vi "Motors Sub 05.vi"(7 "Cluster":T1, 8 "error in":errorcluster, 11 "VISA in":refnum<visa-resource-name>) -> (0 "error out":errorcluster, 3 "VISA out":refnum<visa-resource-name>)   [LabVIEW 2010]
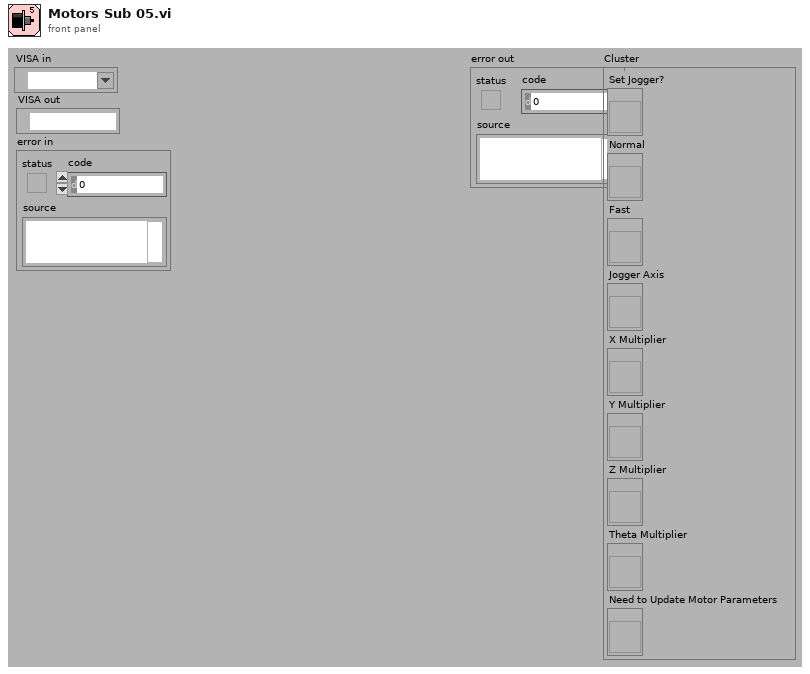
[diagram p1: front panel]
types:
  T1 = cluster{"Set Jogger?":refnum<vi>, "Normal":refnum<vi>, "Fast":refnum<vi>, "Jogger Axis":refnum<vi>, "X Multiplier":refnum<vi>, "Y Multiplier":refnum<vi>, "Z Multiplier":refnum<vi>, "Theta Multiplier":refnum<vi>, "Need to Update Motor Parameters":refnum<vi>}
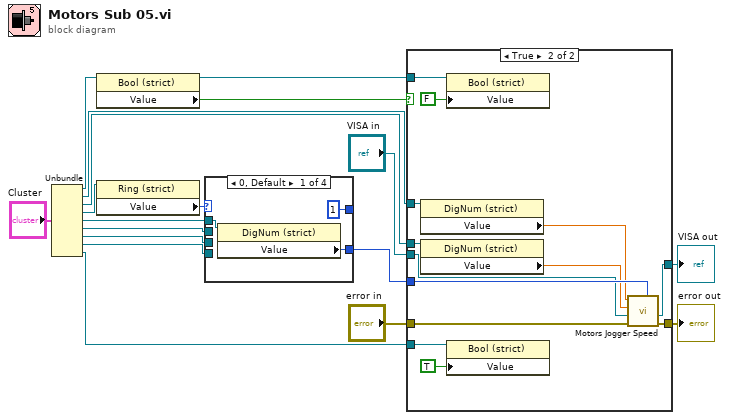
[diagram p0: block diagram]
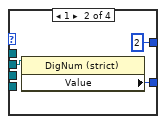
[diagram p2: hidden frame]
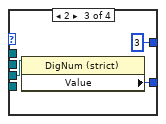
[diagram p3: hidden frame]
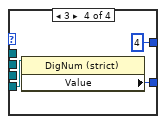
[diagram p4: hidden frame]
diagram:
  n1 = Unbundle("Cluster") -> ("Set Jogger?"=w18:refnum<vi>, "Normal"=w16:refnum<vi>, "Fast"=w15:refnum<vi>, "Jogger Axis"=w12:refnum<vi>, "X Multiplier"=w10:refnum<vi>, "Y Multiplier"=w9:refnum<vi>, "Z Multiplier"=w8:refnum<vi>, "Theta Multiplier"=w7:refnum<vi>, "Need to Update Motor Parameters"=w1:refnum<vi>)
  n2 = property on="Property Node" class="Bool (strict)"(reference=w18) -> (reference out=w14:refnum<vi>, "Value"=w17:bool)  [unwired: 1 in, 1 out]
  n3 = property on="Property Node" class="Ring (strict)"(reference=w12) -> ("Value"=w11:u16)  [unwired: 1 in, 2 out]
  n4 = case shown="0, Default" w11 {
    tunnel: [u32 1 u32 2 u32 3 u32 4] -> _
    tunnel: [w20 w23 w26 w29] -> w13
    tunnel: w10 -> [w19 _ _ _]
    tunnel: w9 -> [_ w22 _ _]
    tunnel: w7 -> [_ _ _ w28]
    tunnel: w8 -> [_ _ w25 _]
    frame 0, Default {
      n5 = property on="Property Node" class="DigNum (strict)"(reference=w19) -> ("Value"=w20:u32)  [unwired: 1 in, 2 out]
    }
    frame 1 {
      n6 = property on="Property Node" class="DigNum (strict)"(reference=w22) -> ("Value"=w23:u32)  [unwired: 1 in, 2 out]
    }
    frame 2 {
      n7 = property on="Property Node" class="DigNum (strict)"(reference=w25) -> ("Value"=w26:u32)  [unwired: 1 in, 2 out]
    }
    frame 3 {
      n8 = property on="Property Node" class="DigNum (strict)"(reference=w28) -> ("Value"=w29:u32)  [unwired: 1 in, 2 out]
    }
  }
  n9 = case shown="True" w17 {
    tunnel: [w32 w45] -> w5
    tunnel: [w31 w43] -> w4
    tunnel: w13 -> [_ w44]
    tunnel: w14 -> [_ w41]
    tunnel: w16 -> [_ w37]
    tunnel: w15 -> [_ w36]
    tunnel: "error in" -> [w32 w35]
    tunnel: "VISA in" -> [w31 w34]
    tunnel: w1 -> [_ w33]
    frame False {
    }
    frame True {
      n10 = property on="Property Node" class="DigNum (strict)"(reference=w37) -> ("Value"=w40:dbl)  [unwired: 1 in, 2 out]
      n11 = property on="Property Node" class="DigNum (strict)"(reference=w36) -> ("Value"=w39:dbl)  [unwired: 1 in, 2 out]
      n12 = property on="Property Node" class="Bool (strict)"(reference=w41, "Value"=FALSE ("Need to Update Motor Parameters")) -> ()  [unwired: 1 in, 2 out]
      n13 = property on="Property Node" class="Bool (strict)"(reference=w33, "Value"=TRUE) -> ()  [unwired: 1 in, 2 out]
      n14 = call "Motors Jogger Speed.vi"("Axis Multiplier"=w44, "error in"=w35, "VISA in"=w34, "Fast Speed (mm or degree/sec)"=w39, "Normal Speed (mm or degree/sec)"=w40) -> ("error out"=w45:errorcluster, "VISA out"=w43:refnum<visa-resource-name>)  [unwired: 5 in]
    }
  }
  "VISA out" <- w4
  "error out" <- w5
